vi "Example NetworkStream Client-Server.vi"() -> ()   [LabVIEW 2013]
uses:
  Connection/Connection.lvclass
  Connection.NetworkStream/Connection.NetworkStream.lvclass
panel:
  out "server connected":bool
  out "client connected":bool
  out "Comm OK":bool
  out "value":dbl
  out "listener error":errorcluster
  out "client session error":errorcluster
  out "server session error":errorcluster
  out "Bytes":u8[](array[numeric]) format="%08b"
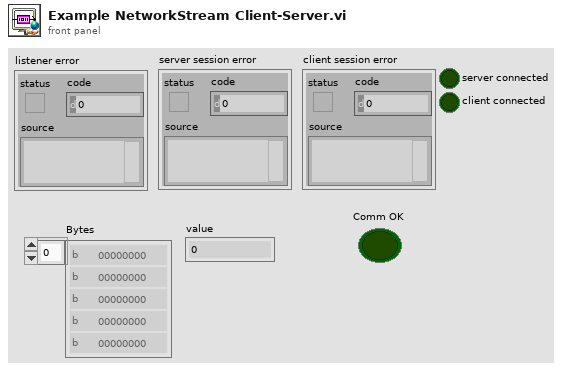
[diagram p1: front panel]
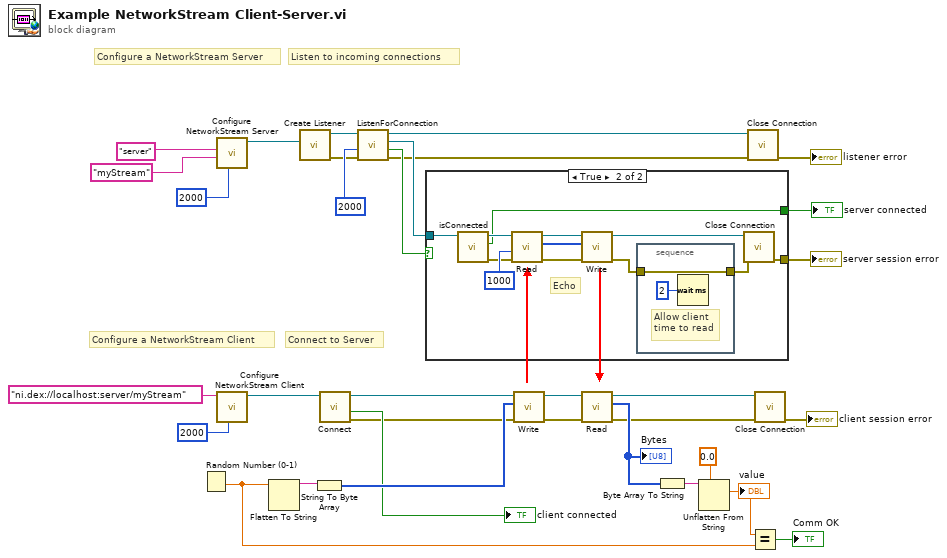
[diagram p0: block diagram]
diagram:
  # "Configure a NetworkStream Client"
  # "Connect to Server"
  # "Listen to incoming connections"
  # "Configure a NetworkStream Server"
  n1 = Random Number (0-1)() -> (number: 0 to 1=w17:dbl)
  n2 = call "Configure NetworkStream Server.vi"("timeout (500 ms)"=2000, "Stream Name"="myStream" ("address (localhost)"), "Context"="server" ("address (localhost)")) -> ("Connection.NetworkStream"=w3:refnum<class "Connection.NetworkStream.lvclass">)  [unwired: 7 in, 1 out]
  n3 = call "Configure NetworkStream Client.vi"("timeout (500 ms)"=2000, "Remote URI"="ni.dex://localhost:server/myStream" ("address (localhost)")) -> ("Connection.NetworkStream"=w14:refnum<class "Connection.NetworkStream.lvclass">)  [unwired: 8 in, 1 out]
  n4 = Flatten To String(anything=w17) -> (data string=w27:string)  [unwired: 3 in, 2 out]
  n5 = call "Create Listener.vi"("Connection Configuration"=w3) -> ("error out"=w30:errorcluster, "Listener"=w33:refnum<class "Connection.lvclass">)  [unwired: 9 in]
  n6 = String To Byte Array(string=w27) -> (unsigned byte array=w26:u8[])
  n7 = call "Connect.vi"("Connection in"=w14) -> ("error out"=w8:errorcluster, "Connection Established"=→"client connected":bool, "Connection out"=w9:refnum<class "Connection.NetworkStream.lvclass">)  [unwired: 8 in]
  n8 = call "ListenForConnection.vi"("error in (no error)"=w30, "timeout (2000 ms)"=2000 ("bytes to read (100)"), "Listener"=w33) -> ("error out"=w1:errorcluster, "New connection"=w13:bool, "Connection"=w15:refnum<class "Connection.lvclass">, "Listener out"=w31:refnum<class "Connection.lvclass">)  [unwired: 5 in]
  n9 = case shown="True" w13 {
    tunnel: [_ w41] -> w2
    tunnel: w15 -> [_ w37]
    tunnel: [_ w34] -> w11
    frame False {
    }
    frame True {
      # "Echo"
      n10 = call "isConnected.vi"("Connection in"=w37) -> ("error out"=w35:errorcluster, "connected"=w34:bool, "Connection out"=w36:refnum<class "Connection.lvclass">)  [unwired: 8 in]
      n11 = call "Read.vi"("error in (no error)"=w35, "timeout (2000 ms)"=1000 ("bytes to read (100)"), "TCPConnection in"=w36) -> ("error out"=w42:errorcluster, "Bytes"=w43:u8[], "TCPConnection out"=w44:refnum<class "Connection.lvclass">)  [unwired: 4 in, 2 out]
      n12 = call "Write.vi"("error in (no error)"=w42, "Bytes"=w43, "Connection in"=w44) -> ("error out"=w39:errorcluster, "Connection"=w40:refnum<class "Connection.lvclass">)  [unwired: 6 in, 1 out]
      n13 = stacked-sequence {
        tunnel: w39 -> [w46]
        tunnel: [w46] -> w38
        frame #0 {
          # "Allow client\ntime to read"
          n14 = Wait (ms)(milliseconds to wait=u32 2) -> ()  [unwired: 1 out]
        }
      }
      n15 = call "Close Connection.vi"("error in (no error)"=w38, "Connection in"=w40) -> ("error out"=w41:errorcluster)  [unwired: 8 in, 1 out]
    }
  }
  "server session error" <- w2
  "server connected" <- w11
  n16 = call "Write.vi"("error in (no error)"=w8, "Bytes"=w26, "Connection in"=w9) -> ("error out"=w28:errorcluster, "Connection"=w29:refnum<class "Connection.NetworkStream.lvclass">)  [unwired: 6 in, 1 out]
  n17 = call "Read.vi"("error in (no error)"=w28, "TCPConnection in"=w29) -> ("error out"=w20:errorcluster, "Bytes"=w25:u8[], "TCPConnection out"=w19:refnum<class "Connection.NetworkStream.lvclass">)  [unwired: 5 in, 2 out]
  "Bytes" <- w25
  n18 = Byte Array To String(unsigned byte array=w25) -> (string=w24:string)
  n19 = Unflatten From String(type=0.0, binary string=w24) -> (value=w18:dbl)  [unwired: 3 in, 2 out]
  "value" <- w18
  n20 = call "Close Connection.vi"("error in (no error)"=w1, "Connection in"=w31) -> ("error out"=→"listener error":errorcluster)  [unwired: 8 in, 1 out]
  n21 = Equal?(x=w18, y=w17) -> (x = y?=→"Comm OK":bool)
  n22 = call "Close Connection.vi"("error in (no error)"=w20, "Connection in"=w19) -> ("error out"=→"client session error":errorcluster)  [unwired: 8 in, 1 out]
